vi "Configure Input Reference.vi"(0 "VISA resource name":refnum<visa-resource-name>, 5 "Platform Slot Number (10)":i16=10 min=-1 max=255, 7 "Input Reference (0:MINimum)":i32(ring) items=["MINimum", "MAXimum", "DEFault", "User Defined Value"], 9 "User Defined Reference Value (12.345)":dbl=12.345 format="%_5g", 11 "error in (no error)":errorcluster) -> (4 "VISA resource name out":refnum<visa-resource-name>, 15 "error out":errorcluster)   [LabVIEW 2018, in "LTB-1.lvlib" / "3150.lvlib"]
doc: "Configures the reference value for the attenuation, in dB for the current wavelength."
uses:
  3150.lvlib
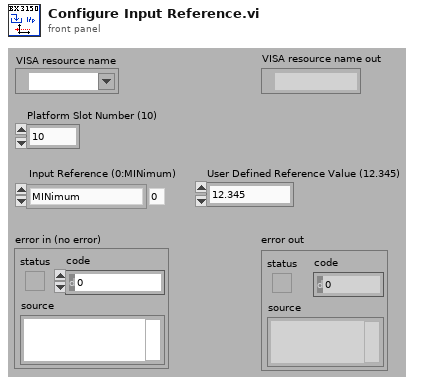
[diagram p1: front panel]
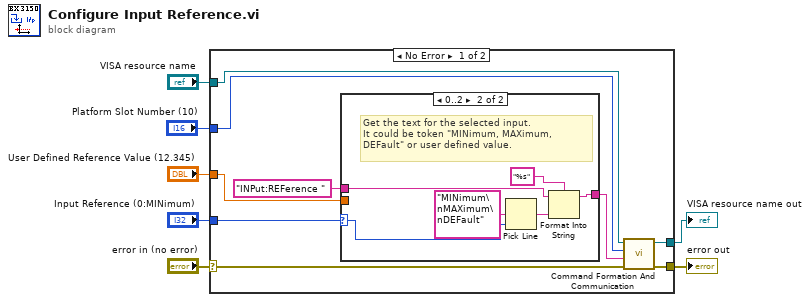
[diagram p0: block diagram]
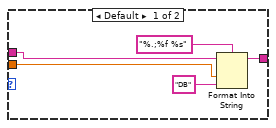
[diagram p2: hidden frame]
diagram:
  n1 = case shown="No Error" "error in (no error)" {
    selector: "error in (no error)" -> [w12 w29]
    tunnel: "VISA resource name" -> [w14 w28]
    tunnel: [w11 w29] -> w5
    tunnel: "Input Reference (0:MINimum)" -> [w9 _]
    tunnel: "Platform Slot Number (10)" -> [w13 _]
    tunnel: [w10 w28] -> w2
    tunnel: "User Defined Reference Value (12.345)" -> [w8 _]
    frame No Error {
      n2 = case shown="0..2" w9 {
        selector: w9 -> [_ w23]
        tunnel: "INPut:REFerence " ("Command") -> [w20 w24]
        tunnel: [w19 w22] -> w15
        tunnel: w8 -> [w18 _]
        frame Default {
          n3 = Format Into String(format string="%.;%f %s", initial string=w20, w18, "DB") -> (resulting string=w19:string)  [unwired: 1 in, 1 out]
        }
        frame 0..2 {
          # "Get the text for the selected input.\nIt could be token \"MINimum, MAXimum,\nDEFault\" or user defined value."
          n4 = Pick Line(multi-line string="MINimum\nMAXimum\nDEFault", line index=w23) -> (output string=w25:string)  [unwired: 1 out]
          n5 = Format Into String(format string="%s", initial string=w24, w25) -> (resulting string=w22:string)  [unwired: 1 in, 1 out]
        }
      }
      n6 = call "Command Formation And Communication.vi"("error in (no error)"=w12, "Command"=w15, "Platform Slot Number"=w13, "VISA resource name"=w14) -> ("error out"=w11:errorcluster, "VISA resource name out"=w10:refnum<visa-resource-name>)  [unwired: 6 out]
    }
    frame Error {
    }
  }
  "VISA resource name out" <- w2
  "error out" <- w5
